vi "Load Hardware.vi"(8 "error in (no error)":errorcluster, 10 "Program only changes":bool=TRUE, 11 "NI Card in":refnum<class "NI Card.lvclass">) -> (0 "error out":errorcluster, 3 "NI Card out":refnum<class "NI Card.lvclass">)   [LabVIEW 2013, in "NI Card.lvclass"]
uses:
  NI Card.lvclass
  NI Card.lvclass/NI Card.ctl
  Globals/Total Time.vi
panel:
  out "error out 2":errorcluster
  out "Last HWI array":T1(array[cluster])
  out "Program?":bool
  out "Names encountered":string[](array[string])
  # "With Clear HW.vi deleting the task,\nProgram only changes will not work with NI cards as currently implemented. i.e. must re-create task every time!\nTherefore, it is disabled and always FALSE."
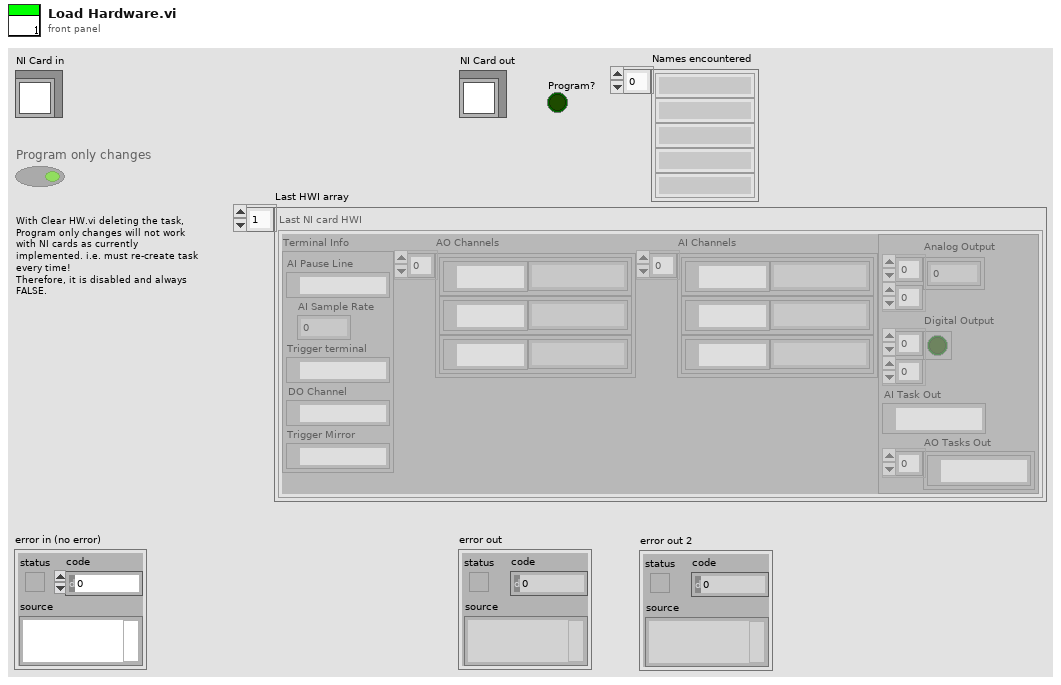
[diagram p1: front panel]
types:
  T1 = cluster{"Terminal Info":cluster{"AI Pause Line":tag, "AI Sample Rate":dbl, "Trigger terminal":tag, "DO Channel":refnum<k21>, "Trigger Mirror":tag}, "AO Channels":cluster{"DAQmx Global Channel":refnum<k21>, "String":string}[], "AI Channels":cluster{"DAQmx Global Channel":refnum<k21>, "String":string}[], "Hardware Image":cluster{"Analog Output ":dbl[][], "Digital Output":bool[][], "AI Task Out":refnum<k21>, "AO Tasks Out":refnum<k21>[]}}[]
  T2 = cluster{"AI Pause Line":tag, "AI Sample Rate":dbl, "Trigger terminal":tag, "DO Channel":refnum<k21>, "Trigger Mirror":tag}
  T3 = cluster{"DAQmx Global Channel":refnum<k21>, "String":string}[]
  T4 = cluster{"Analog Output ":dbl[][], "Digital Output":bool[][], "AI Task Out":refnum<k21>, "AO Tasks Out":refnum<k21>[]}
  T5 = cluster{"Terminal Info":cluster{"AI Pause Line":tag, "AI Sample Rate":dbl, "Trigger terminal":tag, "DO Channel":refnum<k21>, "Trigger Mirror":tag}, "AO Channels":cluster{"DAQmx Global Channel":refnum<k21>, "String":string}[], "AI Channels":cluster{"DAQmx Global Channel":refnum<k21>, "String":string}[], "Hardware Image":cluster{"Analog Output ":dbl[][], "Digital Output":bool[][], "AI Task Out":refnum<k21>, "AO Tasks Out":refnum<k21>[]}}
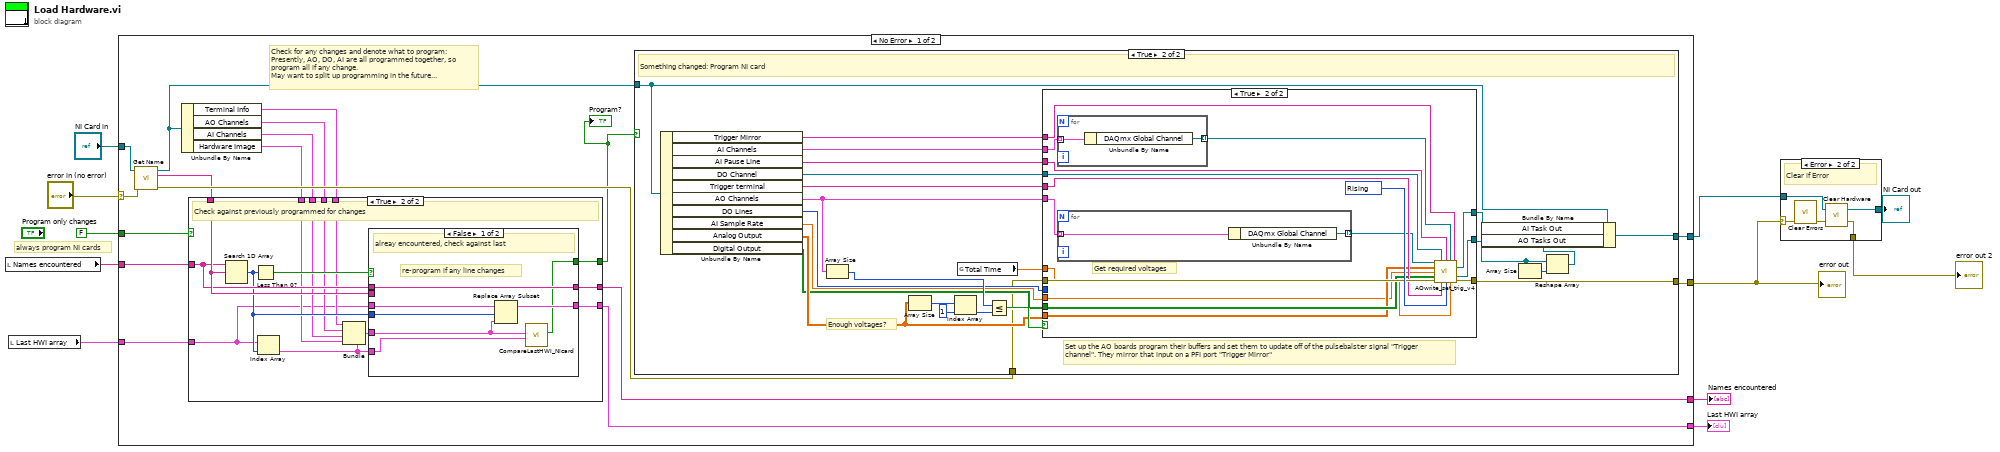
[diagram p0: block diagram]
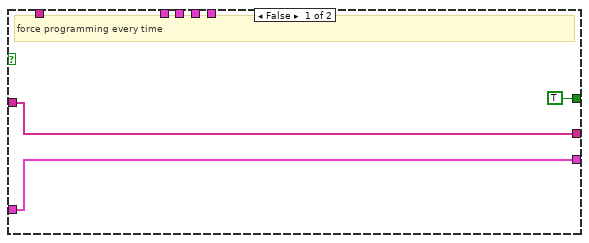
[diagram p3: hidden frame]
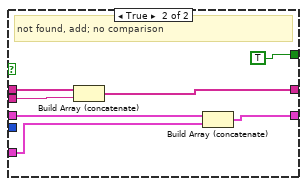
[diagram p4: hidden frame]
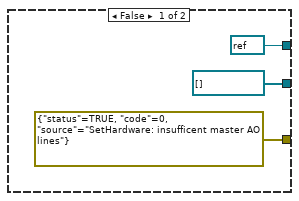
[diagram p6: hidden frame]
diagram:
  # "always program NI cards"
  n1 = local read "Names encountered"() -> (w9:string[])
  n2 = local read "Last HWI array"() -> (w8:T1)
  n3 = case shown="No Error" "error in (no error)" {
    selector: "error in (no error)" -> [w24 w113]
    tunnel: [w28 w113] -> w4
    tunnel: [w27 w112] -> w2
    tunnel: "NI Card in" -> [w26 w112]
    tunnel: FALSE ("Program only changes") -> [w22 _]
    tunnel: w9 -> [w20 w111]
    tunnel: w8 -> [w15 w110]
    tunnel: [w14 w111] -> w7
    tunnel: [w13 w110] -> w6
    frame No Error {
      # "Check for any changes and denote what to program:\nPresently, AO, DO, AI are all programmed together, so\nprogram all if any change.\nMay want to split up programming in the future..."
      n4 = call-dynamic "Get Name.vi"("error in (no error)"=w24, "Device in"=w26) -> ("error out"=w25:errorcluster, "Name"=w21:string, "Device out"=w23:refnum<class "NI Card.lvclass">)  [unwired: 7 in]
      n5 = Unbundle By Name(w23) -> ("Terminal Info"=w19:T2, "AO Channels"=w18:T3, "AI Channels"=w17:T3, "Hardware Image"=w16:T4)
      n6 = case shown="True" w22 {
        tunnel: [TRUE ("Diff?") w45] -> w12
        tunnel: [w31 w44] -> w14
        tunnel: w15 -> [w29 w32]
        tunnel: [w29 w43] -> w13
        tunnel: w19 -> [_ w37]
        tunnel: w21 -> [_ w41]
        tunnel: w20 -> [w31 w40]
        tunnel: w18 -> [_ w36]
        tunnel: w17 -> [_ w35]
        tunnel: w16 -> [_ w34]
        frame False {
          # "force programming every time"
        }
        frame True {
          # "Check against previously programmed for changes"
          n7 = Search 1D Array(1D array=w40, element=w41) -> (index of element=w39:i32)  [unwired: 1 in]
          n8 = Less Than 0?(x=w39) -> (x < 0?=w42:bool)
          n9 = Index Array(array=w32, index=w39) -> (element=w38:T5)
          n10 = Bundle(cluster=w38, "Terminal Info"=w37, "AO Channels"=w36, "AI Channels"=w35, "Hardware Image"=w34) -> (w33:T5)
          n11 = case shown="False" w42 {
            tunnel: w41 -> [_ w58]
            tunnel: w40 -> [w52 w59]
            tunnel: [w52 w57] -> w44
            tunnel: [w46 TRUE] -> w45
            tunnel: w39 -> [w50 _]
            tunnel: [w51 w53] -> w43
            tunnel: w38 -> [w47 _]
            tunnel: w33 -> [w48 w54]
            tunnel: w32 -> [w49 w55]
            frame False {
              # "re-program if any line changes"
              # "alreay encountered, check against last"
              n12 = Replace Array Subset(array=w49, new element=w48, index=w50) -> (w51:T1)
              n13 = call "CompareLastHWI_NIcard.vi"("Last NI card HWI"=w47, "NI card HWI"=w48) -> ("change?"=w46:bool)  [unwired: 9 in]
            }
            frame True {
              # "not found, add; no comparison"
              n14 = Build Array (concatenate)(w59, w58) -> (w57:string[])
              n15 = Build Array (concatenate)(w55, w54) -> (w53:T1)
            }
          }
        }
      }
      "Program?" <- w12
      n16 = case shown="True" w12 {
        tunnel: w25 -> [w60 w70]
        tunnel: [w60 w62] -> w28
        tunnel: [w61 w63] -> w27
        tunnel: w23 -> [w61 w68]
        frame False {
          # "No need to program (Program only changes = TRUE, and Program? = FALSE)"
        }
        frame True {
          # "Enough voltages?"
          # "Set up the AO boards program their buffers and set them to update off of the pulsebalster signal \"Trigger channel\". They mirror that input on a PFI port \"Trigger Mirror\""
          # "Something changed: Program NI card"
          n17 = Unbundle By Name(w68) -> ("Trigger Mirror"=w80:tag, "AI Channels"=w79:T3, "AI Pause Line"=w78:tag, "DO Channel"=w77:refnum<k21>, "Trigger terminal"=w76:tag, "AO Channels"=w75:T3, "DO Lines"=w74:i32, "AI Sample Rate"=w73:dbl, "Analog Output"=w72:dbl[][], "Digital Output"=w71:bool[][])
          n18 = Array Size(array=w75) -> (size(s)=w81:i32)
          n19 = Array Size(array=w72) -> (size(s)=w85:i32[])
          n20 = Index Array(array=w85, index=1 ("Index")) -> (element=w83:i32)
          n21 = global read "Total Time.vi" "Total Time"() -> (w69:dbl)
          n22 = Less Or Equal?(x=w81, y=w83) -> (x <= y?=w82:bool)
          n23 = case shown="True" w82 {
            tunnel: w70 -> [_ w104]
            tunnel: [errorcluster {"status"=TRUE, "code"=0, "source"="SetHardware: insufficent master AO lines"} ("error out") w103] -> w62
            tunnel: [refnum<k21>[] [] w100] -> w65
            tunnel: w75 -> [_ w90]
            tunnel: w72 -> [_ w95]
            tunnel: w76 -> [_ w102]
            tunnel: w71 -> [_ w96]
            tunnel: w77 -> [_ w101]
            tunnel: w79 -> [_ w92]
            tunnel: [refnum<k21> refnum ("task out") w99] -> w67
            tunnel: w69 -> [_ w98]
            tunnel: w80 -> [_ w97]
            tunnel: w74 -> [_ _]
            tunnel: w78 -> [_ w94]
            tunnel: w73 -> [_ w93]
            frame False {
            }
            frame True {
              w105 = 10280 items=["Rising"=10280, "Falling"=10171] ("active edge")
              # "Get required voltages"
              n24 = for {
                tunnel: w92 -> [w109] mode=indexing
                tunnel: [w108] -> w91 mode=indexing
                n25 = Unbundle By Name(w109) -> ("DAQmx Global Channel"=w108:refnum<k21>)
              }
              n26 = for {
                tunnel: w90 -> [w107] mode=indexing
                tunnel: [w106] -> w89 mode=indexing
                n27 = Unbundle By Name(w107) -> ("DAQmx Global Channel"=w106:refnum<k21>)
              }
              n28 = call "AOwrite_set_trig_v4.vi"("AO Channels"=w89, "DO Channel"=w101, "Pause.DigLvl.Src"=w94, "AI Channels"=w91, "Pulse terminal"=w97, "AO Data array"=w95, "AI Sample Rate"=w93, "DO Data array"=w96, "error in"=w104, "Source terminal"=w102, "active edge"=w105, "Total Time"=w98) -> ("AI Task Out"=w99:refnum<k21>, "Tasks Out"=w100:refnum<k21>[], "error out"=w103:errorcluster)  [unwired: 1 out]
            }
          }
          n29 = Array Size(array=w65) -> (size(s)=w64:i32)
          n30 = Reshape Array(w65, w64) -> (w66:refnum<k21>[])
          n31 = Bundle By Name(cluster=w68, "AI Task Out"=w67, "AO Tasks Out"=w66) -> (w63:refnum<class "NI Card.lvclass">)
        }
      }
    }
    frame Error {
    }
  }
  "error out" <- w4
  "Names encountered" <- w7
  "Last HWI array" <- w6
  n32 = case shown="Error" w4 {
    selector: w4 -> [w114 w119]
    tunnel: [w115 w120] -> w3
    tunnel: w2 -> [w115 w117]
    tunnel: [w114 w116] -> w1
    frame No Error {
      # "Pass-through"
    }
    frame Error {
      # "Clear if Error"
      n33 = call <vilib>:"Clear Errors.vi"("error in (no error)"=w119) -> ("error out"=w118:errorcluster)  [unwired: 6 in]
      n34 = call-dynamic "Clear Hardware.vi"("error in (no error)"=w118, "NI Card in"=w117) -> ("error out"=w116:errorcluster, "NI Card out"=w120:refnum<class "NI Card.lvclass">)
    }
  }
  "NI Card out" <- w3
  "error out 2" <- w1
